vi "Teleop.vi"(10 "Match Info":T1={"Autonomous Elapsed Seconds"=0.0, "TeleOp Elapsed Seconds"=0.0, "Disabled Elapsed Seconds"=0.0, "Visited Autonomous"=FALSE, "Visited TeleOp"=FALSE, "Visited Disabled"=FALSE, "Autonomous Settings"={"Autonomous Style"=enum."Independent", "VI Refnum"=refnum}}, 11 "Call Context":T2) -> ()   [LabVIEW 2016]
doc: "This VI is called for each TeleOp packet received from the DS where the robot is not disabled. It is often used to read from the joysticks and update I/O or to update setpoints for timed control loops. It should complete and return within 20 milliseconds or it may miss DS packets."
uses:
  <vilib>/Rock Robotics/WPI/DriverStation/WPI_DriverStationDerivedRobotMode.ctl
  <vilib>/Rock Robotics/WPI/DriverStation/WPI_DriverStationMatch Info.ctl
  <vilib>/Rock Robotics/WPI/Utilities/WPI_GetSetVariantRefNum.vi
  <vilib>/Rock Robotics/Network Tables/NT Write Boolean.vi
  <vilib>/Rock Robotics/Network Tables/NT Write Boolean Array.vi
  <vilib>/Rock Robotics/Network Tables/NT Write Numeric Array.vi
  <vilib>/Rock Robotics/WPI/Solenoid/Deprecated/WPI_SolenoidSetBool.vi
  <vilib>/Rock Robotics/WPI/Ultrasonic/WPI_SonarMB1010AnalogRefNum Registry Get.vi
  <vilib>/Rock Robotics/WPI/Ultrasonic/WPI_SonarMB1010AnalogGetRange.vi
  <vilib>/Rock Robotics/Network Tables/NT Read Number.vi
  <vilib>/Rock Robotics/Network Tables/NT Write Number.vi
panel:
  out "gyro":dbl
  out "sonar distance (inches)":dbl
  out "Encoder Loop 2":string
  out "Encoder Loop":dbl
  out "Encoder Rate":dbl
  out "Encoder State":string
  out "Encoder Direction":string
  out "Distance 2":dbl
  out "Angle 2":dbl
  out "Distance":dbl
  out "Enabled":bool
  out "Compressor Running":bool
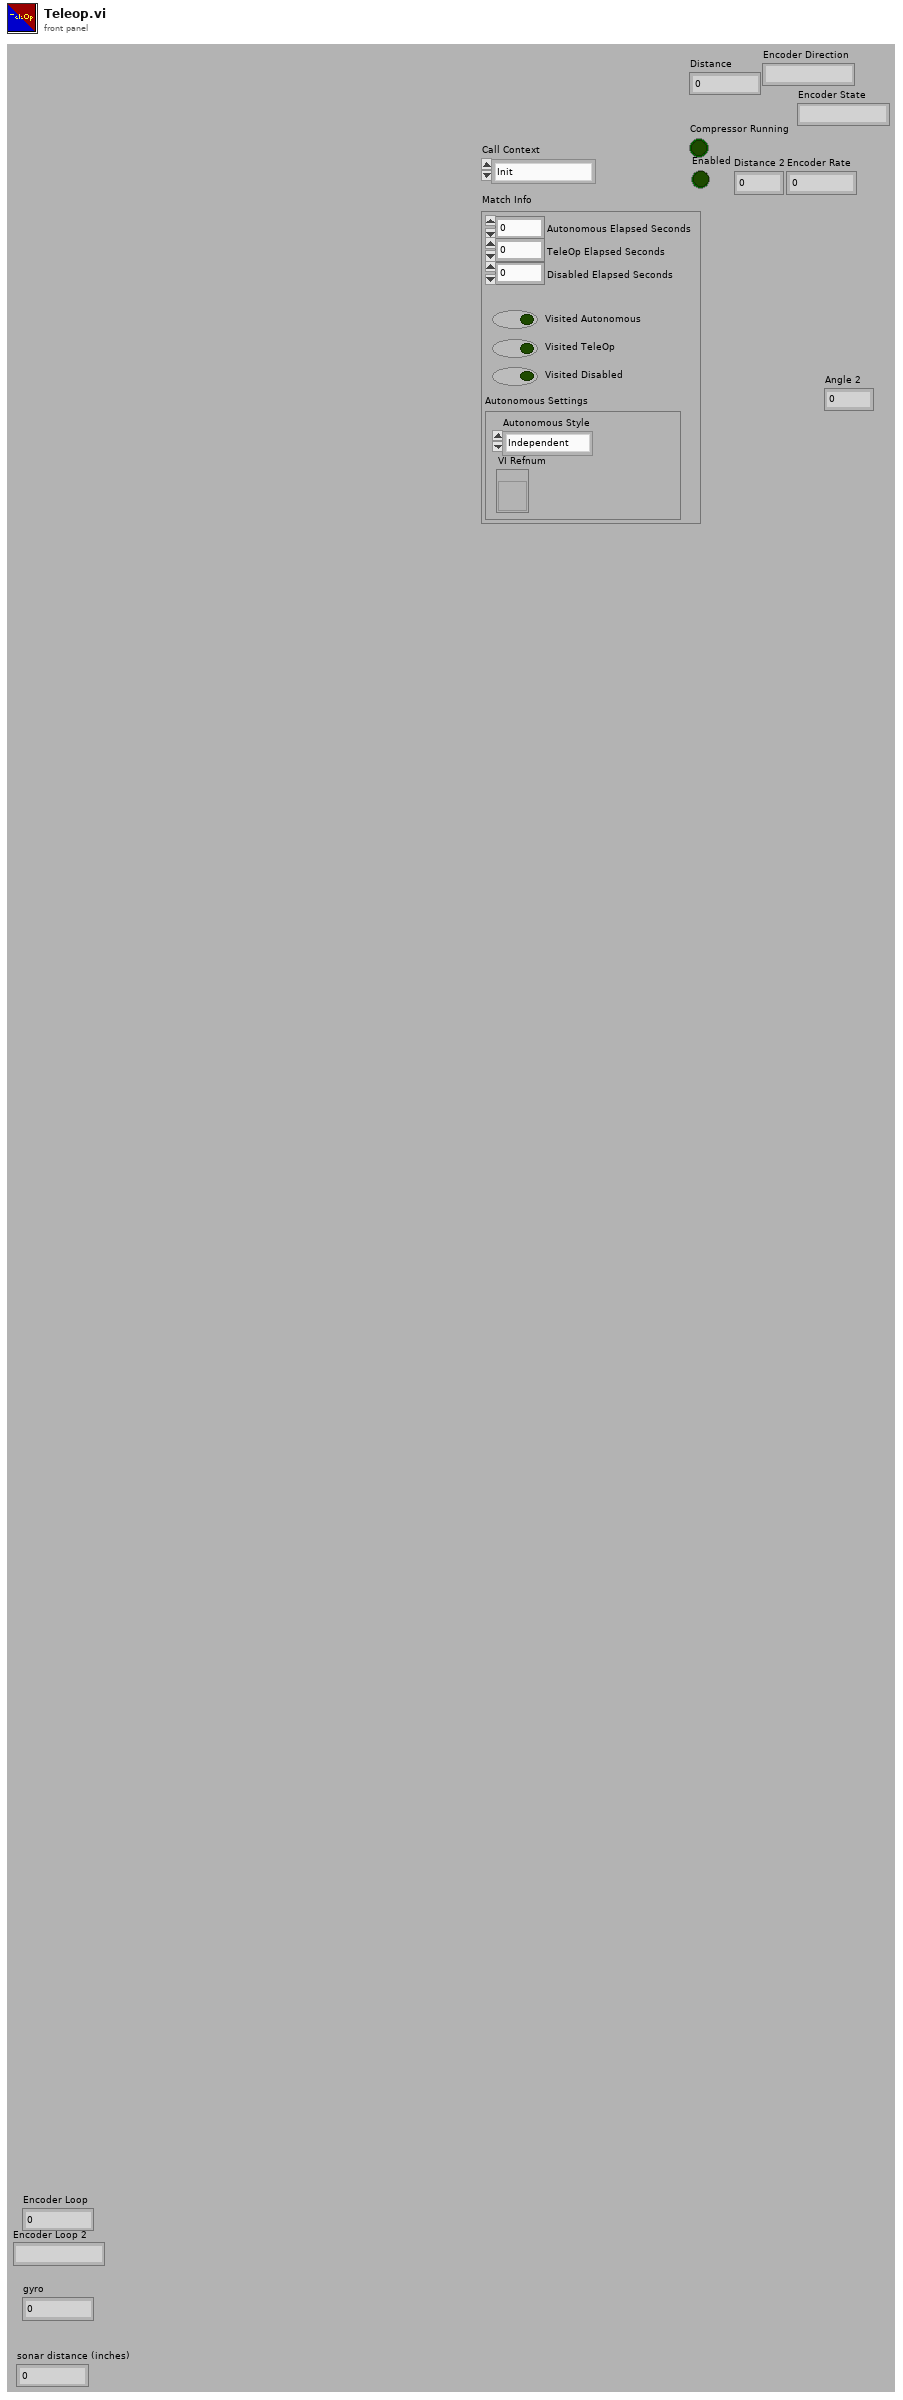
[diagram p1: front panel]
types:
  T1 = typedef "WPI_DriverStationMatch Info.ctl" = cluster{"Autonomous Elapsed Seconds":dbl, "TeleOp Elapsed Seconds":dbl, "Disabled Elapsed Seconds":dbl, "Visited Autonomous":bool, "Visited TeleOp":bool, "Visited Disabled":bool, "Autonomous Settings":cluster{"Autonomous Style":enum16{"Iterative", "Independent"}, "VI Refnum":refnum<vi>}}
  T2 = typedef "WPI_DriverStationDerivedRobotMode.ctl" = enum16{"Init", "Execute", "Stop"}
  T3 = typedef "WPI_EncoderDevRef.ctl" = cluster{"DevStatus":errorcluster, "EncoderIndex":T4, "CounterIndex":T5, "DistancePerCount":dbl, "Decoding Type":T6}
  T4 = typedef "FPGA_EncoderIdx.ctl" = enum8{"Enc 0", "Enc 1", "Enc 2", "Enc 3", "Enc 4", "Enc 5", "Enc 6", "Enc 7", "Invalid"}
  T5 = typedef "FPGA_CounterCtrSystemIndex.ctl" = enum8{"Ctr 0", "Ctr 1", "Ctr 2", "Ctr 3", "Ctr 4", "Ctr 5", "Ctr 6", "Ctr 7", "Invalid"}
  T6 = typedef "WPI_EncoderType.ctl" = enum16{"1x", "2x", "4x"}
  T7 = typedef "WPI_JoystickDevRef.ctl" = cluster{"Device":T8}
  T8 = typedef "WPI_JoystickDeviceEnum.ctl" = enum16{"USB 0", "USB 1", "USB 2", "USB 3", "USB 4", "USB 5"}
  T9 = typedef "WPI_GyroDevRef.ctl" = cluster{"DevStatus":errorcluster, "Analog Channel":T10, "Offset":dbl, "Gain (VoltsPerDegree/Second)":dbl, "Gyro Type":enum16{"Analog", "XRS450"}, "Handle":i32, "SPI Bus":T11, "Device Found":bool, "Sample Rate":dbl, "Calibrate On Open":bool}
  T10 = typedef "FPGA_AIChannel.ctl" = enum8{"AI 0", "AI 1", "AI 2", "AI 3", "AI MXP 0", "AI MXP 1", "AI MXP 2", "AI MXP 3", "Invalid"}
  T11 = typedef "spi_bus.ctl" = enum16{"SPI On-Board, CS0", "SPI On-Board, CS1", "SPI On-Board, CS2", "SPI On-Board, CS3", "SPI MXP", "Invalid"}
  T12 = typedef "WPI_CompressorDevRef.ctl" = cluster{"DevStatus":errorcluster, "Pneumatics Control Module":u8}
  T13 = typedef "WPI_SonarMB1010AnalogDeviceRef.ctl" = cluster{"AIDeviceRef":T14, "Scaling factor (V/in)":dbl, "Average Bits":u8}
  T14 = typedef "WPI_AnalogChannelDevRef.ctl" = cluster{"DevStatus":errorcluster, "Analog Channel":T10}
  T15 = typedef "WPI_SolenoidDevRef.ctl" = cluster{"DevStatus":errorcluster, "Pneumatics Control Module":u8, "Forward Solenoid Channel":T16, "Reverse Solenoid Channel":T16}
  T16 = typedef "WPI_SolenoidChannel.ctl" = enum8{"Solenoid 0", "Solenoid 1", "Solenoid 2", "Solenoid 3", "Solenoid 4", "Solenoid 5", "Solenoid 6", "Solenoid 7", "Invalid"}
  T17 = typedef "WPI_RobotDriveDevRef.ctl" = cluster{"DevStatus":errorcluster, "Motors[]":T18[], "Square Inputs":bool, "Max Output":dbl}
  T18 = typedef "WPI_MotorControlDeviceRef.ctl" = cluster{"DeviceStatus":errorcluster, "Type":T19, "PWM":cluster{"PWM Channel":T20, "DeadBand":T21}, "CAN":cluster{"Device Number":u8, "SetOutput VI Ref":variant, "GetOutput VI Ref":variant, "Enable VI Ref":variant, "Disable VI Ref":variant, "Data":variant}, "Invert":bool}
  T19 = typedef "WPI_MotorControlType.ctl" = enum16{"PWM", "CAN"}
  T20 = typedef "FPGA_DIOPWMChannel.ctl" = enum8{"PWM 0", "PWM 1", "PWM 2", "PWM 3", "PWM 4", "PWM 5", "PWM 6", "PWM 7", "PWM 8", "PWM 9", "PWM MXP 0", "PWM MXP 1", "PWM MXP 2", "PWM MXP 3", "PWM MXP 4", "PWM MXP 5", "PWM MXP 6", "PWM MXP 7", "PWM MXP 8", "PWM MXP 9", "Invalid"}
  T21 = typedef "WPI_PWMDeadband.ctl" = cluster{"Name":string, "maxPositivePwm":i32, "minPositivePwm":i32, "centerPwm":i32, "maxNegativePwm":i32, "minNegativePwm":i32, "angularRange":u16}
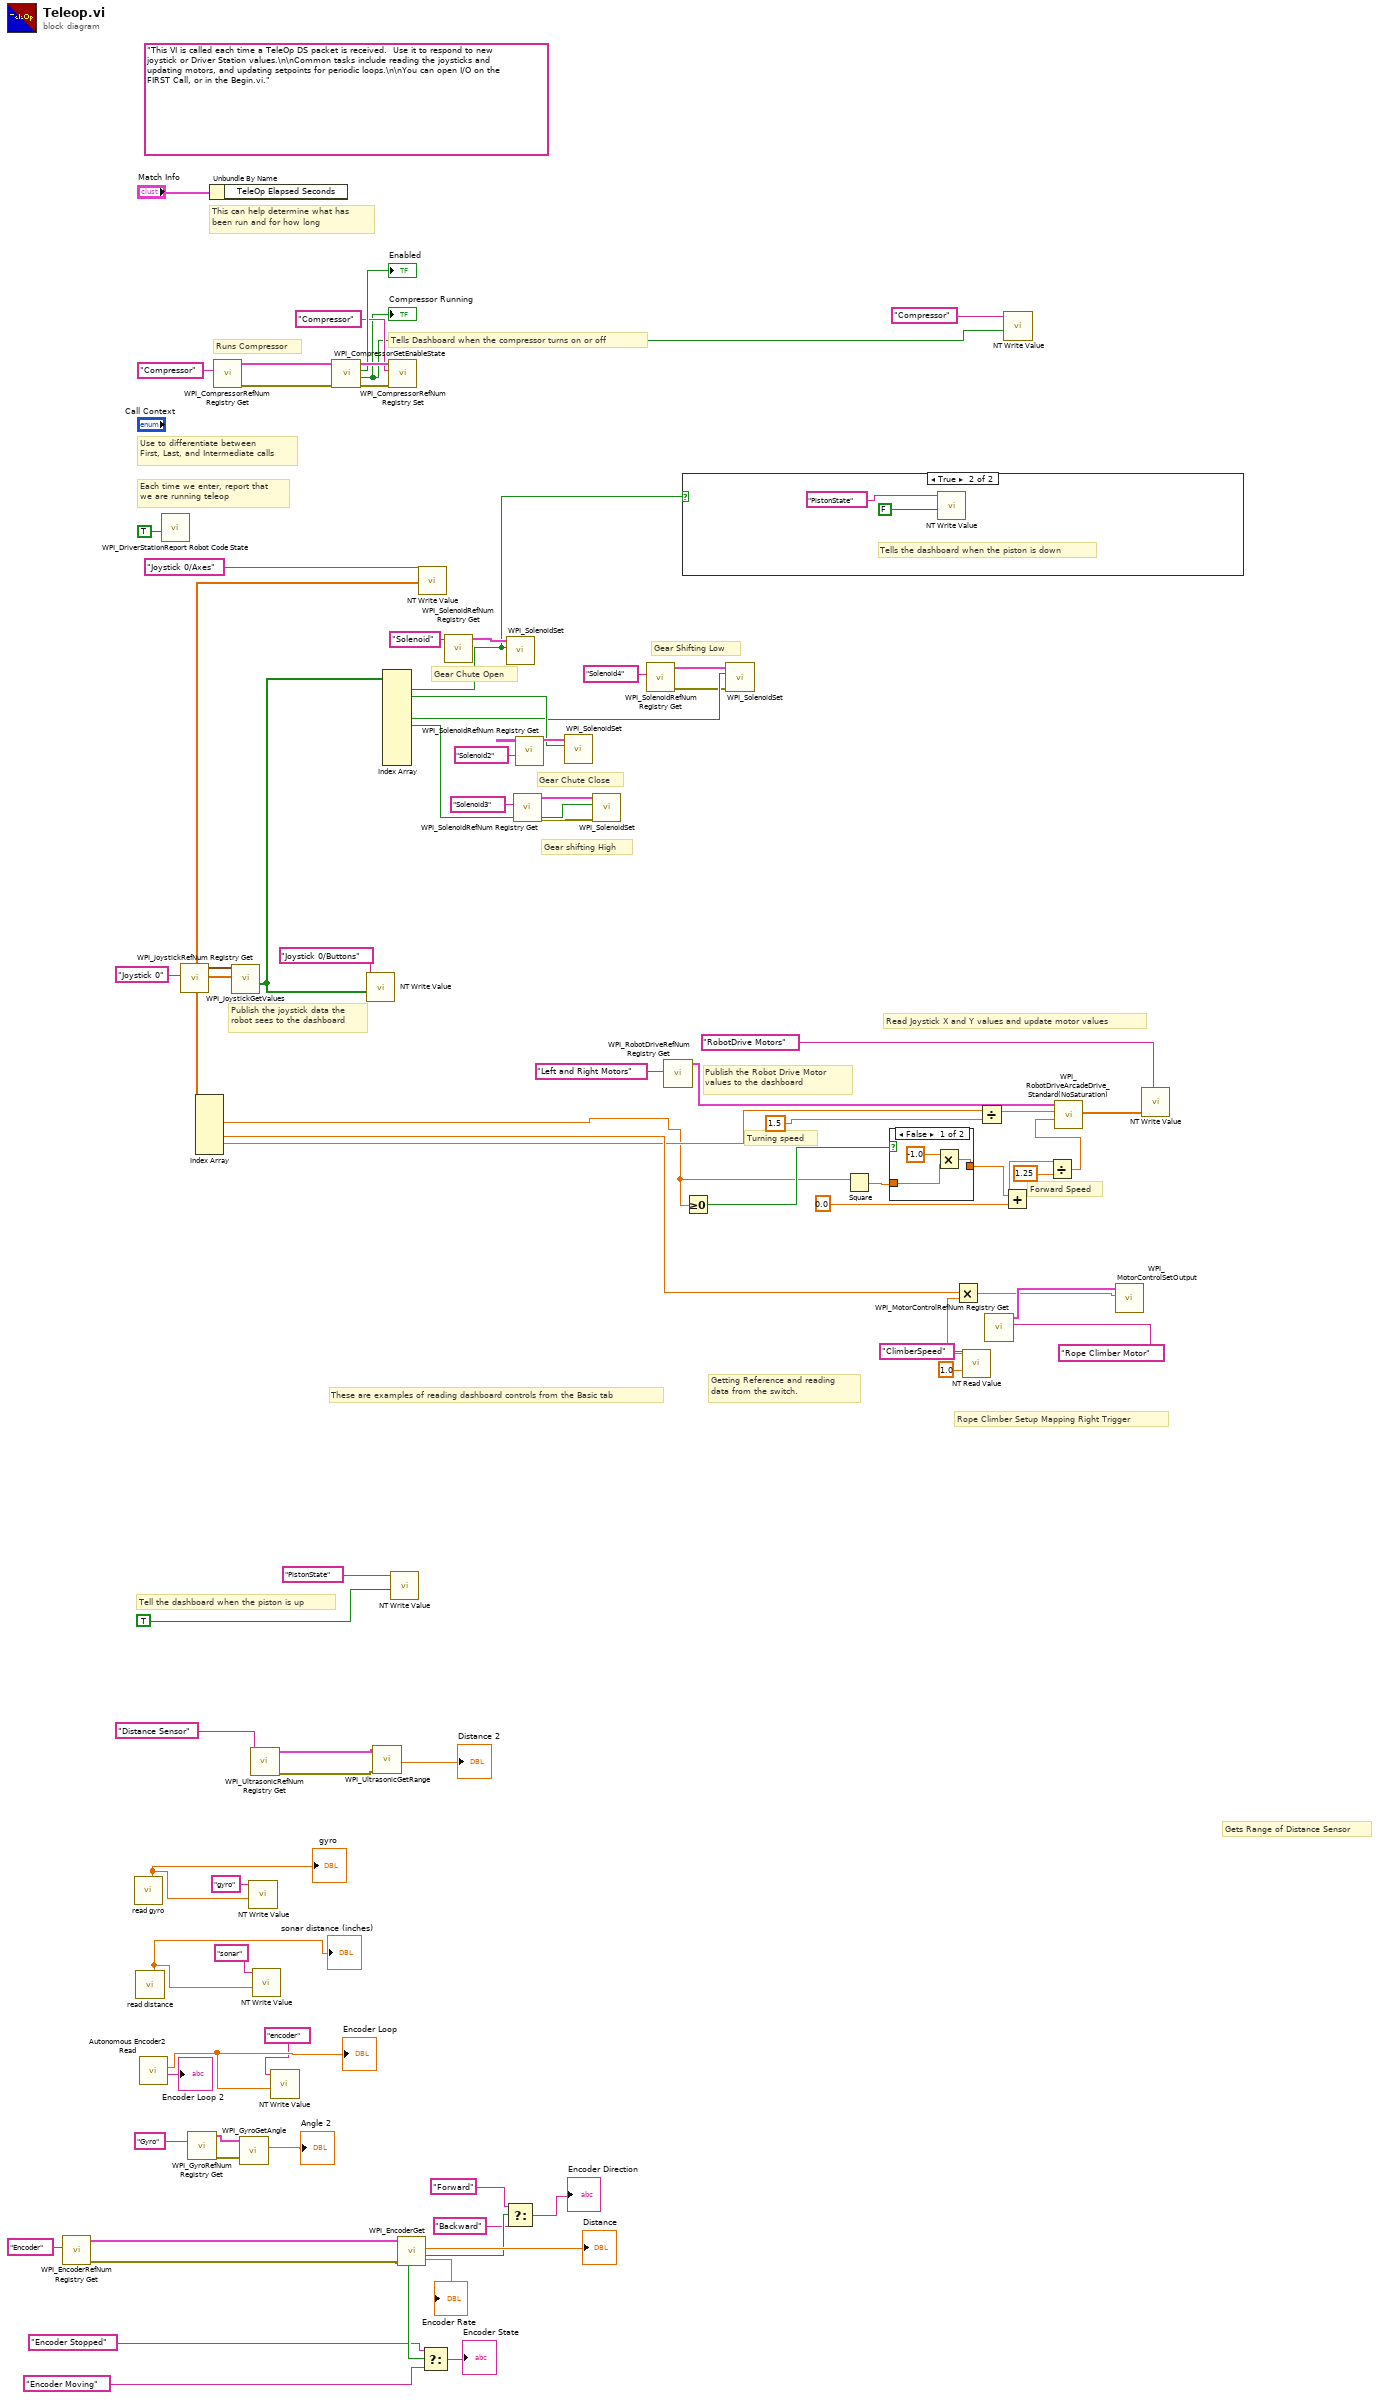
[diagram p0: block diagram]
diagram:
  (unwired) "This VI is called each time a TeleOp DS packet is received.  Use it to respond to new joystick or Driver Station values.\n\nCommon tasks include reading the joysticks and updating motors, and updating setpoints for periodic loops.\n\nYou can open I/O on the FIRST Call, or in the Begin.vi."
  # "Gear Chute Open"
  # "Gear Chute Close"
  # "Gear shifting High"
  # "Gear Shifting Low"
  # "Turning speed"
  # "Forward Speed"
  # "Rope Climber Setup Mapping Right Trigger"
  # "Gets Range of Distance Sensor"
  # "Getting Reference and reading \ndata from the switch."
  # "Tell the dashboard when the piston is up"
  # "Publish the joystick data the\nrobot sees to the dashboard"
  # "Publish the Robot Drive Motor\nvalues to the dashboard"
  # "Read Joystick X and Y values and update motor values"
  # "Tells Dashboard when the compressor turns on or off"
  # "Runs Compressor"
  # "These are examples of reading dashboard controls from the Basic tab"
  # "Each time we enter, report that\nwe are running teleop"
  # "Use to differentiate between\nFirst, Last, and Intermediate calls"
  # "This can help determine what has\nbeen run and for how long"
  n1 = call <vilib>:"WPI_EncoderRefNum Registry Get.vi"("refnum name"="Encoder") -> ("error out"=w49:errorcluster, "EncoderDevRef"=w50:T3)  [unwired: 9 in]
  n2 = call "read gyro.vi"() -> ("Angle 2"=w22:dbl)  [unwired: 10 in, 1 out]
  "gyro" <- w22
  n3 = call "read distance.vi"() -> ("Distance 2"=w20:dbl)  [unwired: 10 in, 1 out]
  "sonar distance (inches)" <- w20
  n4 = call "Autonomous Encoder2 Read.vi"() -> ("Encoder Direction"=→"Encoder Loop 2":string, "Encoder Distance"=w17:dbl)  [unwired: 9 in, 1 out]
  "Encoder Loop" <- w17
  n5 = call <vilib>:"WPI_DriverStationReport Robot Code State.vi"("TeleOp"=TRUE ("Autonomous")) -> ()  [unwired: 10 in, 1 out]
  n6 = call <vilib>:"WPI_JoystickRefNum Registry Get.vi"("refnum name"="Joystick 0") -> ("JoystickDevRef"=w69:T7)  [unwired: 1 in, 9 out]
  n7 = call <vilib>:"WPI_GyroRefNum Registry Get.vi"("refnum name"="Gyro") -> ("error out"=w44:errorcluster, "GyroDevRef"=w45:T9)  [unwired: 9 in]
  n8 = Unbundle By Name("Match Info") -> ()  [unwired: 1 out]
  n9 = call <vilib>:"WPI_CompressorRefNum Registry Get.vi"("refnum name"="Compressor") -> ("error out"=w79:errorcluster, "CompressorDevRef"=w81:T12)  [unwired: 9 in]
  n10 = call <vilib>:"WPI_JoystickGetValues.vi"("JoystickDevRef"=w69) -> ("Buttons"=w63:bool[], "Axes"=w66:dbl[])  [unwired: 6 in, 3 out]
  n11 = Index Array(array=w66) -> (element #2=w15:dbl, element #4=w54:dbl, element #5=w30:dbl)  [unwired: 6 in, 3 out]
  n12 = call <vilib>:"WPI_GyroGetAngle.vi"("error in"=w44, "GyroDevRef"=w45) -> ("Angle"=→"Angle 2":dbl)  [unwired: 5 in, 4 out]
  n13 = call-poly <vilib>:"NT Write Value.vi"("Numeric"=w22, "Name"="gyro") -> ()  [unwired: 9 in, 1 out]
  n14 = call-poly <vilib>:"WPI_UltrasonicRefNum Registry Get.vi"("refnum name"="Distance Sensor") -> ("error out"=w40:errorcluster, "SonarMB1010AnalogDevRef"=w42:T13)  [unwired: 9 in]
  n15 = call-poly <vilib>:"NT Write Value.vi"("Numeric"=w20, "Name"="sonar") -> ()  [unwired: 9 in, 1 out]
  n16 = call-poly <vilib>:"NT Write Value.vi"("Numeric"=w17, "Name"="encoder") -> ()  [unwired: 9 in, 1 out]
  n17 = call <vilib>:"WPI_CompressorGetEnableState.vi"("error in (no error)"=w79, "CompressorDevRef"=w81) -> ("error out"=w78:errorcluster, "Compressor Running"=w73:bool, "Enabled"=→"Enabled":bool, "CompressorDevRef"=w80:T12)  [unwired: 6 in]
  "Compressor Running" <- w73
  n18 = call-poly <vilib>:"NT Write Value.vi"("Boolean Array"=w63, "Name"="Joystick 0/Buttons") -> ()  [unwired: 9 in, 1 out]
  n19 = call-poly <vilib>:"WPI_UltrasonicGetRange.vi"("error in"=w40, "SonarMB1010AnalogDevRef"=w42) -> ("Distance"=→"Distance 2":dbl)  [unwired: 7 in, 2 out]
  n20 = Index Array(array=w63) -> (element #1=w57:bool, element #2=w58:bool, element #5=w7:bool, element #6=w8:bool)  [unwired: 11 in, 7 out]
  n21 = call <vilib>:"WPI_CompressorRefNum Registry Set.vi"("error in (no error)"=w78, "refnum name"="Compressor", "CompressorDevRef"=w80) -> ()  [unwired: 7 in, 2 out]
  n22 = call-poly <vilib>:"NT Write Value.vi"("Boolean"=TRUE, "Name"="PistonState") -> ()  [unwired: 9 in, 1 out]
  n23 = call <vilib>:"WPI_EncoderGet.vi"("error in (no error)"=w49, "EncoderDevRef"=w50) -> ("Direction"=w39:bool, "Distance"=→"Distance":dbl, "Rate"=→"Encoder Rate":dbl, "Stopped"=w35:bool)  [unwired: 4 in, 2 out]
  n24 = call-poly <vilib>:"NT Write Value.vi"("Numeric Array"=w66, "Name"="Joystick 0/Axes") -> ()  [unwired: 9 in, 1 out]
  n25 = Select(t="Encoder Stopped", s=w35, f="Encoder Moving") -> (s? t:f=→"Encoder State":string)
  n26 = call <vilib>:"WPI_SolenoidRefNum Registry Get.vi"("refnum name"="Solenoid") -> ("SolenoidDevRef"=w59:T15)  [unwired: 9 in, 1 out]
  n27 = call-poly <vilib>:"WPI_SolenoidSet.vi"("Value"=w57, "SolenoidDevRef"=w59) -> ()  [unwired: 8 in, 2 out]
  n28 = Select(t="Forward", s=w39, f="Backward") -> (s? t:f=→"Encoder Direction":string)
  n29 = call <vilib>:"WPI_SolenoidRefNum Registry Get.vi"("refnum name"="Solenoid3") -> ("error out"=w1:errorcluster, "SolenoidDevRef"=w3:T15)  [unwired: 9 in]
  n30 = call <vilib>:"WPI_SolenoidRefNum Registry Get.vi"("refnum name"="Solenoid2") -> ("SolenoidDevRef"=w61:T15)  [unwired: 9 in, 1 out]
  n31 = call-poly <vilib>:"WPI_SolenoidSet.vi"("Value"=w58, "SolenoidDevRef"=w61) -> ()  [unwired: 8 in, 2 out]
  n32 = call-poly <vilib>:"WPI_SolenoidSet.vi"("error in (no error)"=w1, "Value"=w8, "SolenoidDevRef"=w3) -> ()  [unwired: 7 in, 2 out]
  n33 = call <vilib>:"WPI_SolenoidRefNum Registry Get.vi"("refnum name"="Solenoid4") -> ("error out"=w4:errorcluster, "SolenoidDevRef"=w6:T15)  [unwired: 9 in]
  n34 = call <vilib>:"WPI_RobotDriveRefNum Registry Get.vi"("refnum name"="Left and Right Motors") -> ("RobotDriveDevRef"=w71:T17)  [unwired: 1 in, 9 out]
  n35 = case shown="True" w57 {
    frame False {
    }
    frame True {
      # "Tells the dashboard when the piston is down"
      n36 = call-poly <vilib>:"NT Write Value.vi"("Boolean"=FALSE, "Name"="PistonState") -> ()  [unwired: 9 in, 1 out]
    }
  }
  n37 = Greater Or Equal To 0?(x=w15) -> (x >= 0?=w25:bool)
  n38 = call-poly <vilib>:"WPI_SolenoidSet.vi"("error in (no error)"=w4, "Value"=w7, "SolenoidDevRef"=w6) -> ()  [unwired: 7 in, 2 out]
  n39 = Square(x=w15) -> (x^2=w24:dbl)
  n40 = case shown="False" w25 {
    tunnel: w24 -> [w88 w89]
    tunnel: [w86 w89] -> w23
    frame False {
      n41 = Multiply(x=-1.0, y=w88) -> (x*y=w86:dbl)
    }
    frame True {
    }
  }
  n42 = call-poly <vilib>:"NT Read Value.vi"("Default Value"=1.0, "Name"="ClimberSpeed") -> ("Numeric"=w11:dbl)  [unwired: 8 in, 1 out]
  n43 = Multiply(x=w54, y=w11) -> (x*y=w10:dbl)
  n44 = Divide(x=w30, y=1.5) -> (x/y=w52:dbl)
  n45 = call <vilib>:"WPI_MotorControlRefNum Registry Get.vi"("refnum name"="Rope Climber Motor") -> ("MotorControlDevRef"=w13:T18)  [unwired: 9 in, 1 out]
  n46 = Add(x=w23, y=0.0) -> (x+y=w27:dbl)
  n47 = call-poly <vilib>:"NT Write Value.vi"("Boolean"=w73, "Name"="Compressor") -> ()  [unwired: 9 in, 1 out]
  n48 = Divide(x=w27, y=1.25) -> (x/y=w26:dbl)
  n49 = call <vilib>:"WPI_RobotDriveArcadeDrive_Standard(NoSaturation).vi"("Y axis value"=w26, "X axis value"=w52, "RobotDriveDevRef"=w71) -> ("Motor Values"=w65:dbl[])  [unwired: 1 in, 7 out]
  n50 = call <vilib>:"WPI_MotorControlSetOutput.vi"("Output"=w10, "MotorControlDevRef"=w13) -> ()  [unwired: 7 in, 3 out]
  n51 = call-poly <vilib>:"NT Write Value.vi"("Numeric Array"=w65, "Name"="RobotDrive Motors") -> ()  [unwired: 9 in, 1 out]
